vi "Model Initial Values - Set Inport Channel Default.vi"(8 "error in":errorcluster, 10 "Default Value":dbl, 11 "Item Ref in":T1 format="%.0x") -> (0 "error out":errorcluster, 3 "Item Ref out":T1 format="%.0x")   [LabVIEW 2011, in "Model Initial Values Custom Device.lvlib"]
uses:
  Model Initial Values Custom Device.lvlib
  <vilib>/NI Veristand/Custom Device API/Custom Device Item Ref.ctl
  NationalInstruments.VeriStand.SystemStorage
  <vilib>/NI Veristand/Custom Device API/Custom Device API.lvlib
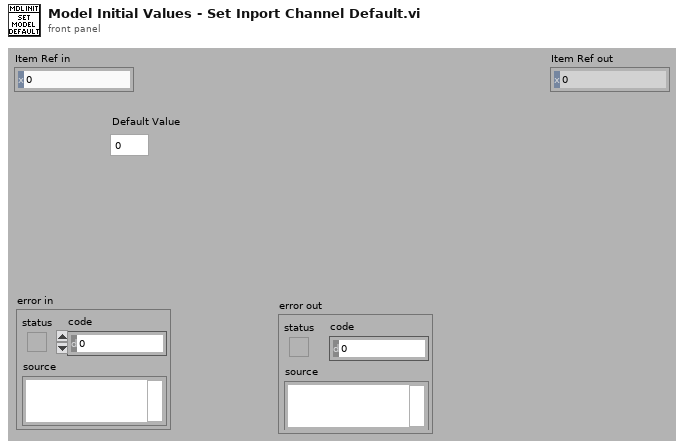
[diagram p1: front panel]
types:
  T1 = typedef "Custom Device API.lvlib/Custom Device Item Ref.ctl" = u64
  T2 = typedef "Custom Device API.lvlib/Custom Device Pointer.ctl" = refnum<k24>
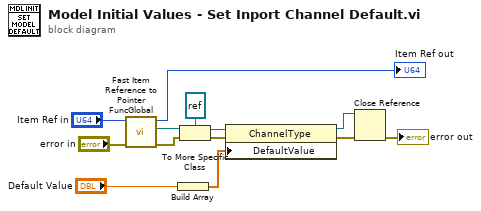
[diagram p0: block diagram]
diagram:
  n1 = call "Fast Item Reference to Pointer FuncGlobal.vi"("error in (no error)"="error in", "Item Ref in"="Item Ref in") -> ("error out"=w1:errorcluster, "Node Pointer"=w2:T2, "Item Ref out"=→"Item Ref out":T1)  [unwired: 6 in, 1 out]
  n2 = Build Array("Default Value") -> (w10:dbl[])
  n3 = To More Specific Class(target class=refnum<k24> refnum ("BaseNodeType"), reference=w2, error in=w1) -> (specific class reference=w12:refnum<k24>, error out=w13:errorcluster)
  n4 = property class="ChannelType"(reference=w12, error in=w13, "DefaultValue"=w10) -> (reference out=w8:refnum<k24>, error out=w7:errorcluster)
  n5 = Close Reference(reference=w8, error in (no error)=w7) -> (error out=→"error out":errorcluster)
